vi "Save Data (SubVI).vi"(10 "queue out":refnum<queue>, 11 "队列输入":refnum<queue>) -> (3 "队列输出":refnum<queue>)   [LabVIEW 2019, in "SubVI.lvlib"]
uses:
  SubVI.lvlib
  config.ctl
  Instrument.ctl
  lib/QDInstrument.dll
  <vilib>/NI/Modbus Library/API/Master/Modbus Master.lvclass
  <vilib>/Utility/file.llb/Write Delimited Spreadsheet (string).vi
panel:
  # "(真是通道1，假是通道2)"
  # "(真是通道1，假是通道2)"
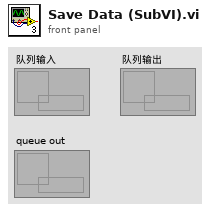
[diagram p1: front panel]
types:
  T1 = typedef "config.ctl" = cluster{"initialize":string, "6221":cluster{"6221 Resource":refnum<visa-resource-name>, "Delta status":bool}, "7001":cluster{"Ch":bool}, "SR830+6221":cluster{"source":u16, "阻抗":dbl, "量程入 4":i32, "量程入 3":i32, "量程入 2":i32, "量程入 1":i32, "电流":dbl, "SR830 2":bool, "SR830 3":bool, "SR830 4":bool, "SR830 1":bool, "VISA 1":refnum<visa-resource-name>, "VISA 2":refnum<visa-resource-name>, "VISA 3":refnum<visa-resource-name>, "VISA 4":refnum<visa-resource-name>, "量程":enum16{"量程每次测量会判定", "量程不变为设定值"}}, "2400":cluster{"2400":bool, "VISA":refnum<visa-resource-name>}, "ch":cluster{"ch str":string, "ch1":bool, "ch2":bool, "布尔":bool}, "error":bool, "数据文件路径":path, "log":cluster{"log路径":path, "log interval":dbl}, "Instrument":T2}
  T2 = typedef "Instrument.ctl" = cluster{"335 Resource":refnum<visa-resource-name>, "Input (0:A)":u16, "Instrument Type":i32, "quantum design":refnum<k24>, "Heater Output (1:1)":u16, "335state":refnum<vi>, "semaphore":T3, "TCP master instance":refnum<class "Modbus Master.lvclass">}
  T3 = typedef "Semaphore RefNum" = refnum<k1>
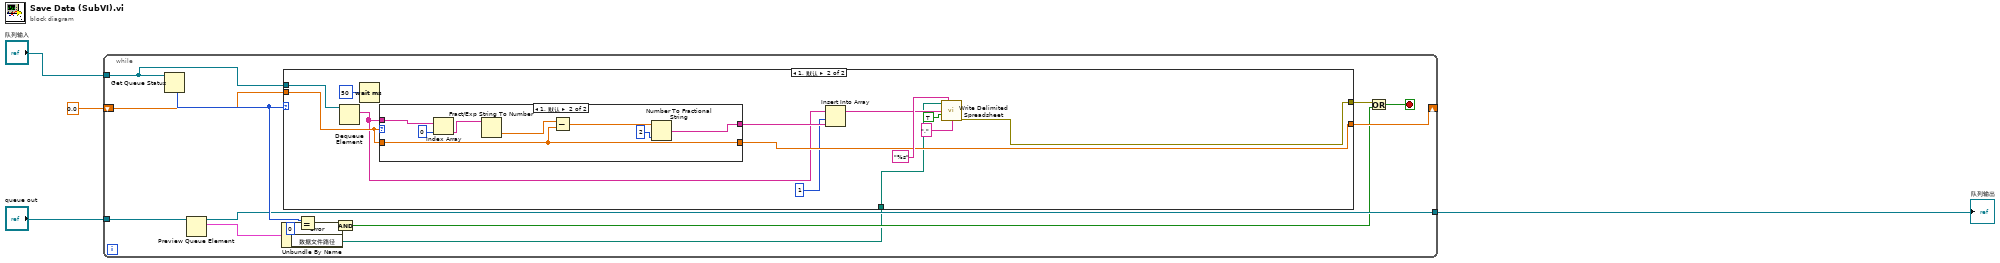
[diagram p0: block diagram]
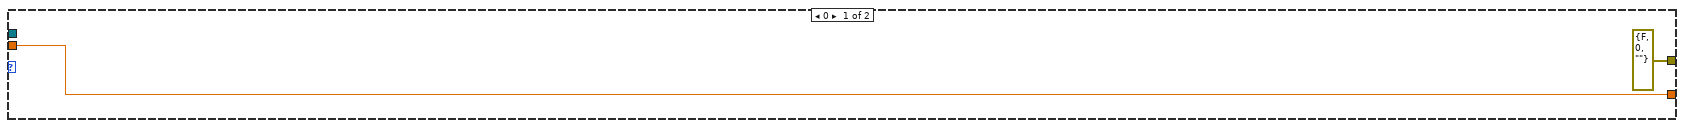
[diagram p2: hidden frame]
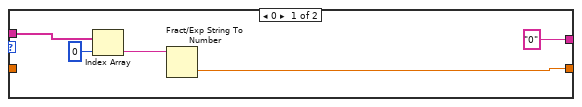
[diagram p3: hidden frame]
diagram:
  n1 = while {
    tunnel: "队列输入" -> [w18]
    tunnel: "queue out" -> [w17]
    tunnel: [w13] -> w1
    shift-right: [w12] -> _
    shift-left: 0.0 ("数值") -> [w11]
    stop <- w8 stop-if-true
    n2 = Get Queue Status(queue=w18) -> (# elements in queue=w16:i32)  [unwired: 2 in, 7 out]
    n3 = Preview Queue Element(queue=w17) -> (queue out=w13:refnum<queue>, element=w7:T1)  [unwired: 2 in, 2 out]
    n4 = Unbundle By Name(w7) -> ("error"=w6:bool, "数据文件路径"=w5:path)
    n5 = case shown="1, 默认" w16 {
      tunnel: w18 -> [_ w29]
      tunnel: [w20 w28] -> w12
      tunnel: w11 -> [w20 w25]
      tunnel: [errorcluster {"status"=FALSE, "code"=0, "source"=""} ("error out") w24] -> w9
      tunnel: w5 -> [_ w21]
      frame 0 {
      }
      frame 1, Default {
        n6 = Dequeue Element(queue=w29) -> (element=w23:string[])  [unwired: 2 in, 3 out]
        n7 = Wait (ms)(milliseconds to wait=u32 50 ("等待时间（毫秒）")) -> ()  [unwired: 1 out]
        n8 = case shown="1, 默认" w25 {
          tunnel: w23 -> [w38 w45]
          tunnel: [w34 w39] -> w28
          tunnel: w25 -> [_ w39]
          tunnel: ["0" w41] -> w27
          frame 0 {
            n9 = Index Array(array=w38, index=0 ("索引")) -> (element=w35:string)
            n10 = Fract/Exp String To Number(string=w35) -> (number=w34:dbl)  [unwired: 3 in, 1 out]
          }
          frame 1, Default {
            n11 = Index Array(array=w45, index=0 ("索引")) -> (element=w44:string)
            n12 = Fract/Exp String To Number(string=w44) -> (number=w40:dbl)  [unwired: 3 in, 1 out]
            n13 = Subtract(x=w40, y=w39) -> (x-y=w43:dbl)
            n14 = Number To Fractional String(number=w43, precision (6)=i16 2 ("精度(6)")) -> (F-format string=w41:string)  [unwired: 2 in]
          }
        }
        n15 = Insert Into Array(array=w23, index=1 ("索引"), new element=w27) -> (w22:string[])
        n16 = call-poly <vilib>:"Write Delimited Spreadsheet.vi"("file path (dialog if empty)"=w21, "format (%s)"="%s" ("format (%.3f)"), "1D data"=w22, "append to file? (new file:F)"=TRUE, "delimiter (\\t)"="," ("delimiter (\\t)")) -> ("error out"=w24:errorcluster)  [unwired: 9 in, 1 out]
      }
    }
    n17 = Equal?(x=w16, y=0) -> (x = y?=w14:bool)
    n18 = And(x=w14, y=w6) -> (x .and. y?=w10:bool)
    n19 = Or(x=w9, y=w10) -> (x .or. y?=w8:bool)
  }
  "队列输出" <- w1
